vi "Acquire Image.vi"(8 "Error In":errorcluster, 11 "Camera In":T2="cam1") -> (0 "Error Out":errorcluster, 2 "Image":T1(plugin-control), 3 "Camera Out":T2="cam1")   [LabVIEW 2018]
uses:
  <vilib>/userdefined/High Color/IMAQdx.ctl
  <vilib>/vision/driver/NI_Vision_Acquisition_Software.lvlib
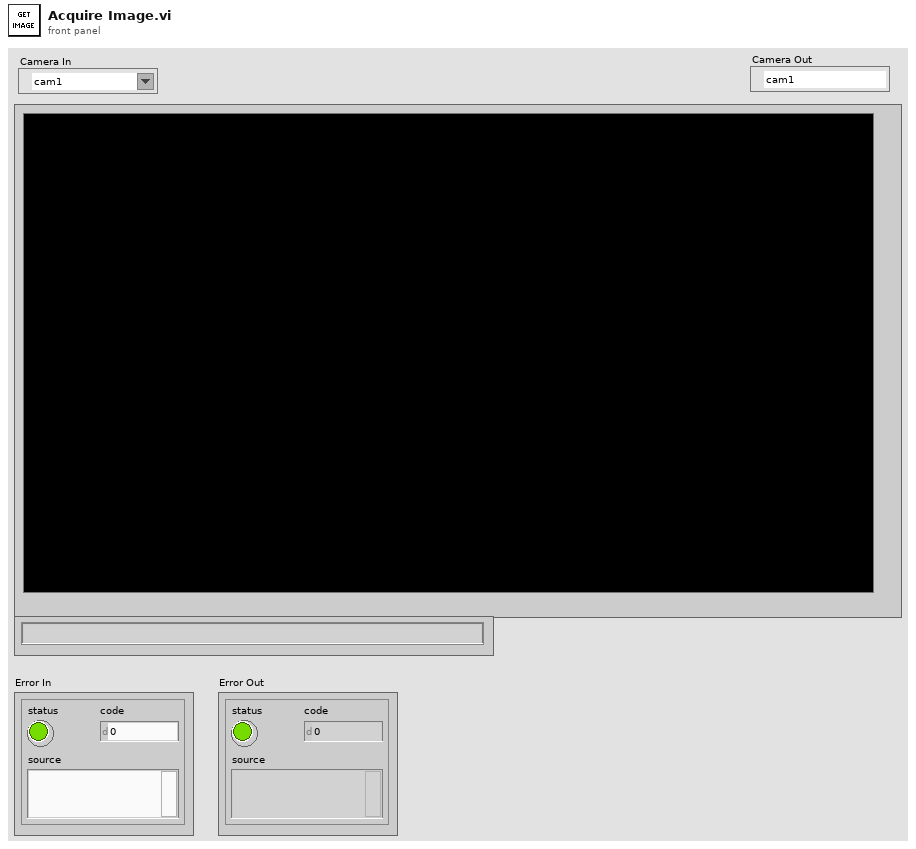
[diagram p1: front panel]
types:
  T1 = typedef "IMAQ Image.ctl" = refnum<image>
  T2 = typedef "IMAQdx.ctl" = refnum<k21>
  T3 = typedef "Image Type" = u32
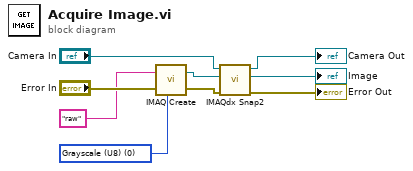
[diagram p0: block diagram]
diagram:
  w1 = T3 0 items=["Grayscale (U8)", "Grayscale (I16)", "Grayscale (SGL)", "Complex (CSG)", "RGB (U32)", "HSL (U32)", "RGB (U64)", "Grayscale (U16)"] ("Image Type")
  n1 = call "IMAQ Create"("Image Name"="raw", "Image Type"=w1, "error in (no error)"="Error In") -> ("New Image"=w7:T1, "error out"=w5:errorcluster)  [unwired: 2 in]
  n2 = call <vilib>:"IMAQdx Snap2.vi"("error in"=w5, "Image In"=w7, "Session In"="Camera In") -> ("error out"=→"Error Out":errorcluster, "Image Out"=→"Image":T1, "Session Out"=→"Camera Out":T2)  [unwired: 6 in]
